vi "principal.vi"() -> ()   [LabVIEW 2010]
uses:
  <vilib>/addons/internet/NI_InternetTK_Common_VIs.lvlib
panel:
  out "status":bool
  out "Localizar Instrumento":u8(slide) scale=0.0..200.0
  out "Execução do ensaio":u8(slide) scale=0.0..100.0
  in  "inicio_time":string
  out "Contador_sim":bool
  out "Siave_sim":bool
  out "Excel._Workbook":refnum<k7>
  out "error out":errorcluster
  out "Excel._Worksheet":refnum<k7>
  in  "Tab k":T1(tab) caption="Tab Control 2"
  in  "Table 12000":string[][](table)
  in  "Table 20000":string[][](table)
  in  "Table 32000":string[][](table)
  in  "Table 40000":string[][](table)
  in  "Table 50000":string[][](table)
  in  "Table 65000":string[][](table)
  in  "Iniciar 2":bool
  in  "Iniciar":bool
  out "Rh %":dbl format="%.2g"
  out "Temp. ºC":dbl format="%.2g"
  in  "Patrimônio":string
  in  "Técnico executor":string
  out "k_list":i32[](array[numeric])=[1000, 2000, 4000, 8000, 15000, 40000]
  out "Vel_list":dbl[](array[numeric])
  out "nk * nVel":i32
  out "Serial disponivel":refnum<visa-resource-name>
  out "Velocidade":dbl
  out "Iteração atual":dbl
  out "Iterações":dbl
  out "Vmax":dbl
  out "Vmin":dbl
  out "k":dbl
  out "Freq. Atual":dbl format="%#.10g"
  out "Freq. Teórica":dbl format="%#.9g"
  out "Contador":bool
  out "Motover":bool
  # "Calibração do Motover"
  # "Equipamento Conectado"
  # "Parâmetros"
  # "Leitura Atual"
  # "simulação?"
  # "Identificação"
  # "Ensaio iniciado em:"
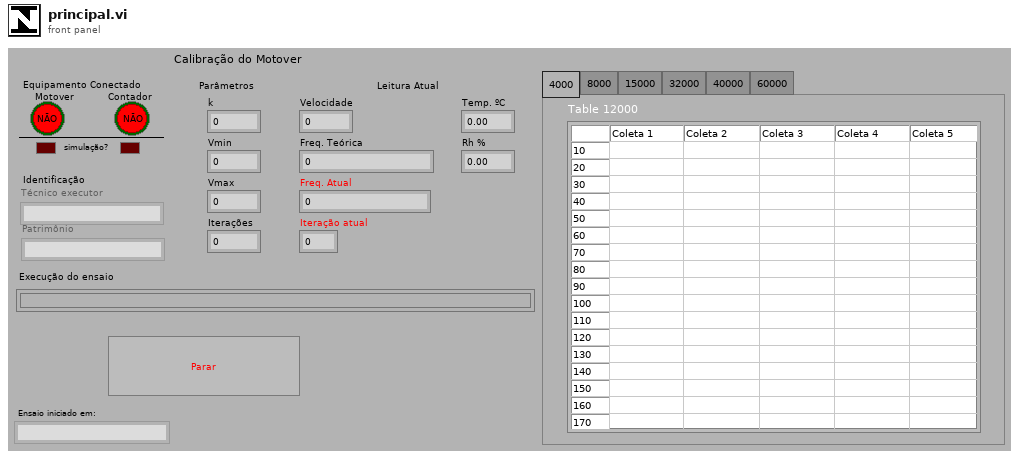
[diagram p1: front panel]
types:
  T1 = enum32{"4000", "8000", "15000", "32000", "40000", "60000"}
  T2 = enum8{"Enabled", "Disabled", "Disabled and Grayed Out"}
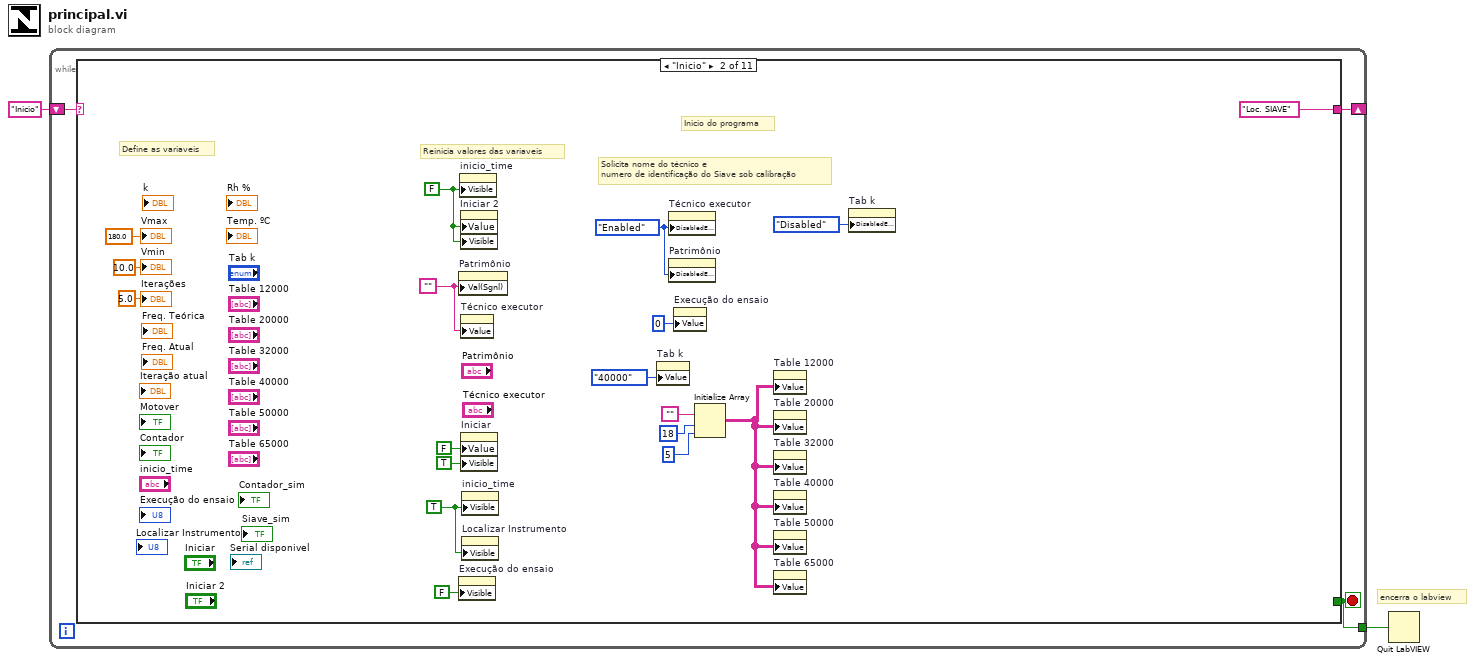
[diagram p0: block diagram]
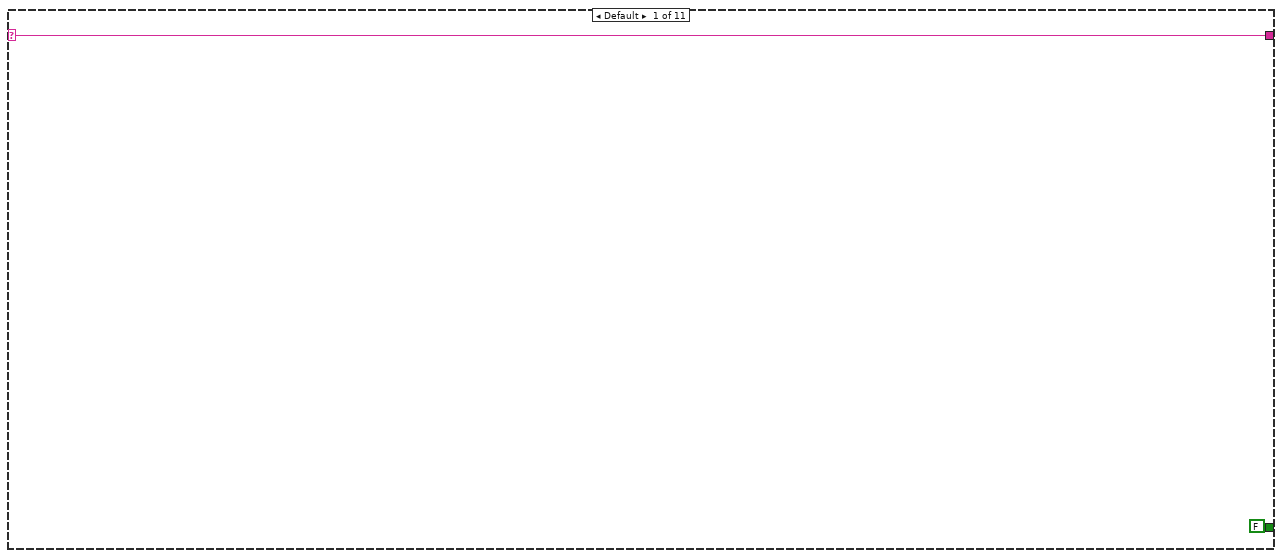
[diagram p2: hidden frame]
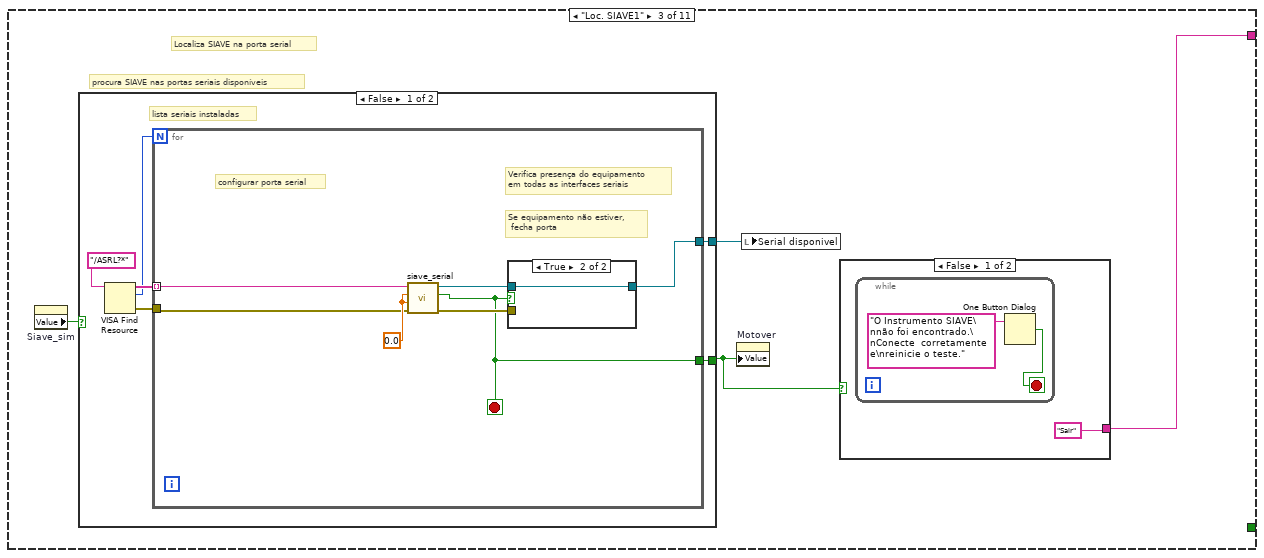
[diagram p3: hidden frame]
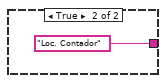
[diagram p4: hidden frame]
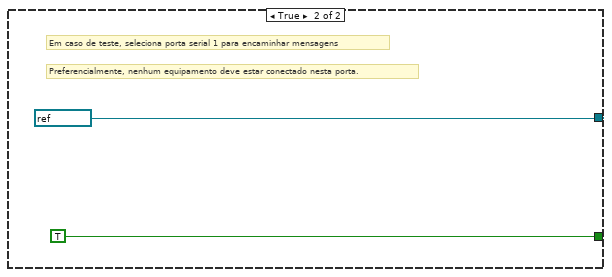
[diagram p6: hidden frame]
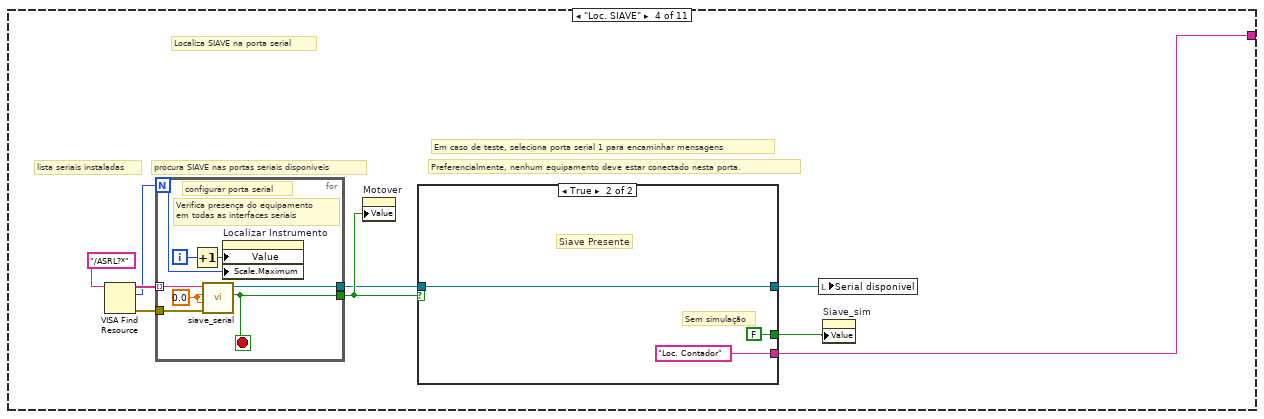
[diagram p7: hidden frame]
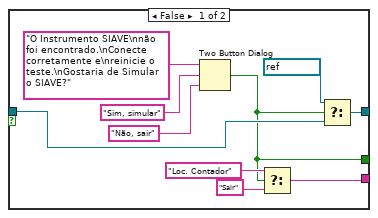
[diagram p8: hidden frame]
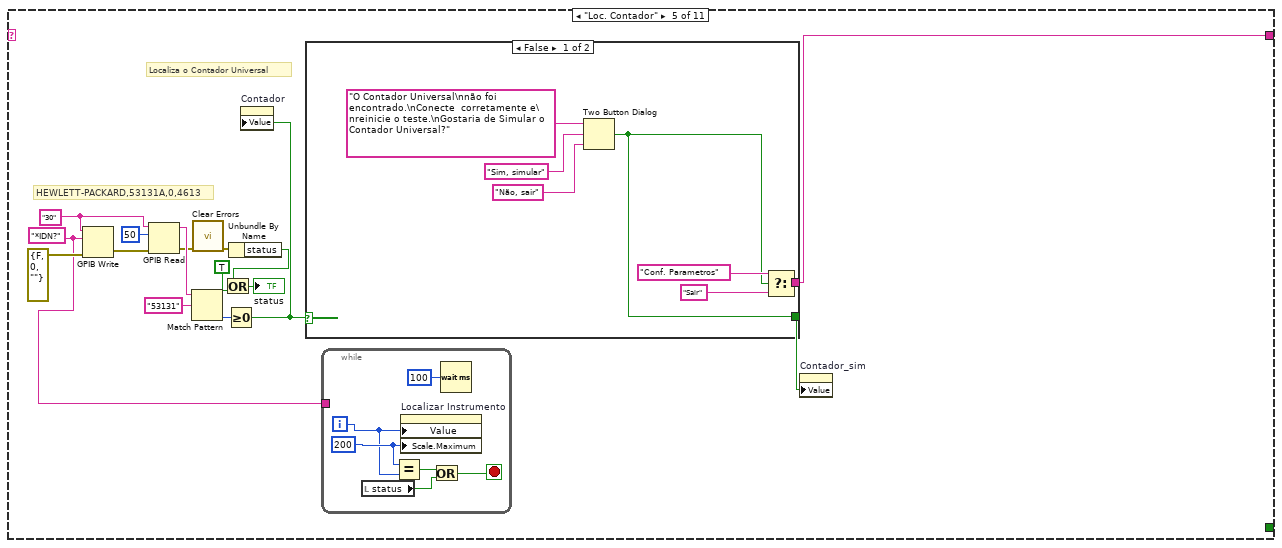
[diagram p9: hidden frame]
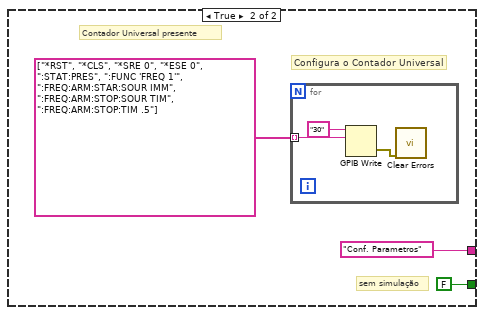
[diagram p10: hidden frame]
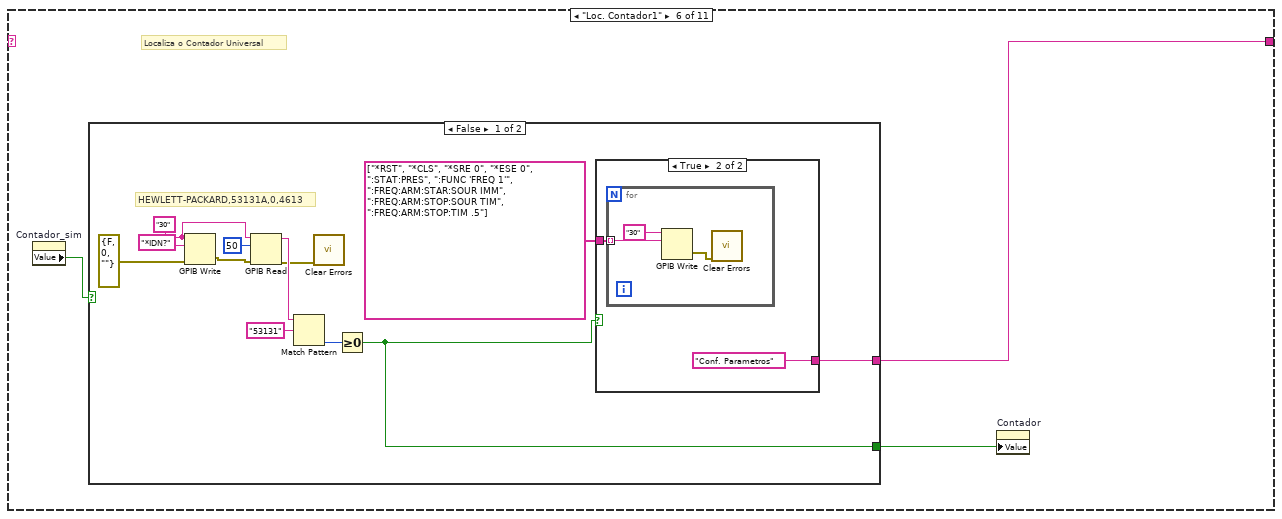
[diagram p11: hidden frame]
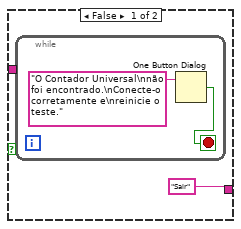
[diagram p12: hidden frame]
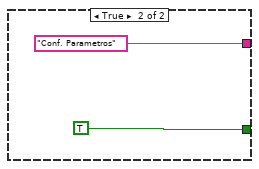
[diagram p13: hidden frame]
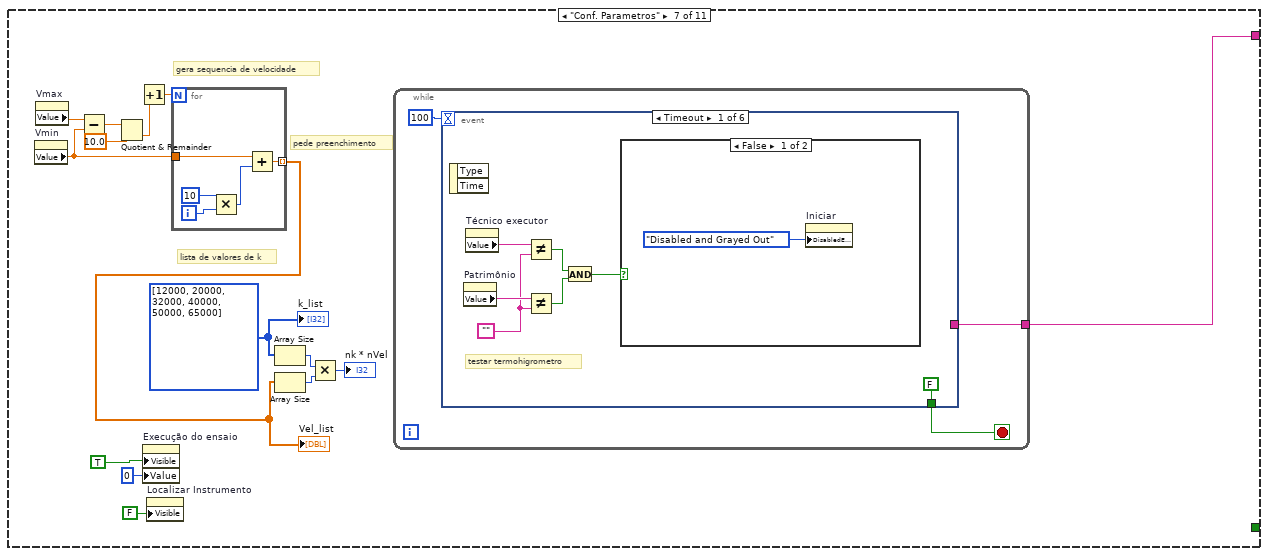
[diagram p14: hidden frame]
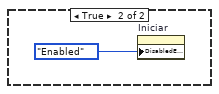
[diagram p15: hidden frame]
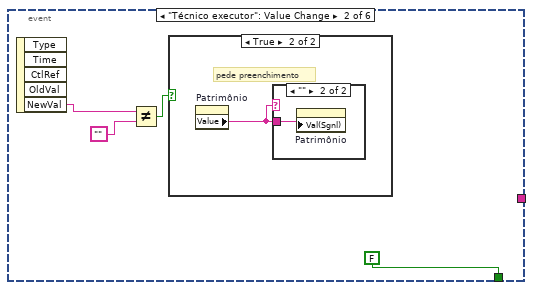
[diagram p16: hidden frame]
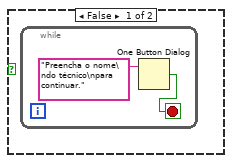
[diagram p17: hidden frame]
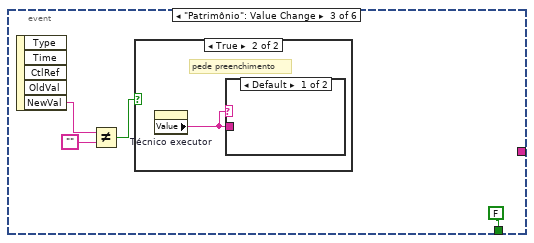
[diagram p19: hidden frame]
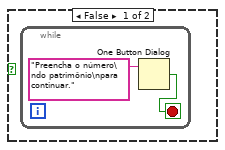
[diagram p20: hidden frame]
diagram:
  # "encerra o labview"
  n1 = while {
    shift-right: [w4] -> _
    shift-left: "Inicio" -> [w5]
    tunnel: [w3] -> w1
    stop <- w3 stop-if-true
    n2 = case shown="\"Inicio\"" w5 {
      selector: w5 -> [w6 _ _ _ _ _ _ _ _ _ _]
      tunnel: [FALSE _ _ _ _ _ _ _ _ _ TRUE] -> w3
      tunnel: [w6 "Loc. SIAVE" w27 w57 w85 w116 w143 "Coletar" w246 "Sair" "Sair"] -> w4
      frame Default {
      }
      frame "Inicio" {
        w9 = TRUE
        w20 = T2."Enabled" ("Disabled")
        w18 = FALSE ("Visible")
        w21 = ""
        # "Reinicia valores das variaveis"
        # "Solicita nome do técnico e\nnumero de identificação do Siave sob calibração"
        # "Define as variaveis"
        # "Inicio do programa"
        n3 = property on="Patrimônio" class="Str"("Val(Sgnl)"=w21) -> ()  [unwired: 2 in, 2 out]
        n4 = property on="Execução do ensaio" class="Slide (strict)"("Visible"=FALSE) -> ()  [unwired: 2 in, 2 out]
        n5 = property on="inicio_time" class="Str"("Visible"=w18) -> ()  [unwired: 2 in, 2 out]
        n6 = property on="Iniciar 2" class="Bool (strict)"("Value"=w18, "Visible"=w18) -> ()  [unwired: 2 in, 2 out]
        n7 = property on="Técnico executor" class="Str"("Value"=w21) -> ()  [unwired: 2 in, 2 out]
        n8 = property on="Iniciar" class="Bool (strict)"("Value"=FALSE ("Iniciar"), "Visible"=TRUE) -> ()  [unwired: 2 in, 2 out]
        n9 = property on="inicio_time" class="Str"("Visible"=w9) -> ()  [unwired: 2 in, 2 out]
        n10 = property on="Localizar Instrumento" class="Slide (strict)"("Visible"=w9) -> ()  [unwired: 2 in, 2 out]
        n11 = property on="Tab k" class="TabCtl (strict)"("Value"=T1."40000" ("Tab k")) -> ()  [unwired: 2 in, 2 out]
        n12 = property on="Técnico executor" class="Str"("DisabledEnum"=w20) -> ()  [unwired: 2 in, 2 out]
        n13 = property on="Patrimônio" class="Str"("DisabledEnum"=w20) -> ()  [unwired: 2 in, 2 out]
        n14 = property on="Execução do ensaio" class="Slide (strict)"("Value"=u8 0 ("Execução do ensaio")) -> ()  [unwired: 2 in, 2 out]
        n15 = Initialize Array("", 18, 5 ("dimension size")) -> (w12:string[][])
        n16 = property on="Table 12000" class="Tbl (strict)"("Value"=w12) -> ()  [unwired: 2 in, 2 out]
        n17 = property on="Table 20000" class="Tbl (strict)"("Value"=w12) -> ()  [unwired: 2 in, 2 out]
        n18 = property on="Table 32000" class="Tbl (strict)"("Value"=w12) -> ()  [unwired: 2 in, 2 out]
        n19 = property on="Table 40000" class="Tbl (strict)"("Value"=w12) -> ()  [unwired: 2 in, 2 out]
        n20 = property on="Table 50000" class="Tbl (strict)"("Value"=w12) -> ()  [unwired: 2 in, 2 out]
        n21 = property on="Table 65000" class="Tbl (strict)"("Value"=w12) -> ()  [unwired: 2 in, 2 out]
        n22 = property on="Tab k" class="TabCtl (strict)"("DisabledEnum"=T2."Disabled" ("Disabled")) -> ()  [unwired: 2 in, 2 out]
        "Vmin" <- 10.0 ("Vmin")
        "Vmax" <- 180.0 ("Vmax")
        "Iterações" <- 5.0 ("Iterações")
      }
      frame "Loc. SIAVE1" {
        # "procura SIAVE nas portas seriais disponíveis"
        # "Localiza SIAVE na porta serial"
        n23 = property on="Siave_sim" class="Bool (strict)"() -> ("Value"=w29:bool)  [unwired: 2 in, 2 out]
        n24 = case shown="False" w29 {
          tunnel: [w38 refnum<visa-resource-name> "COM1" ("VISA resource name out")] -> w26
          tunnel: [w37 TRUE] -> w28
          frame False {
            # "lista seriais instaladas"
            n25 = VISA Find Resource(11:"/ASRL?*" ("expression (\"?*\")")) -> (0:w35:errorcluster, 2:w34:u32, 3:w36:string[])  [unwired: 2 in]
            n26 = for {
              N: w34 -> [_]
              tunnel: w36 -> [w41] mode=indexing
              tunnel: [w45] -> w37
              tunnel: [w44] -> w38
              tunnel: w35 -> [w40]
              stop <- w45 stop-if-true
              w42 = 0.0 ("velocidade")
              # "Se equipamento não estiver,\n fecha porta"
              # "configurar porta serial"
              # "Verifica presença do equipamento\nem todas as interfaces seriais"
              n27 = call "siave_serial.vi"("error in (no error)"=w40, "velocidade"=w42, "k"=w42, "VISA resource name"=w41) -> ("error out"=w46:errorcluster, "ok"=w45:bool, "VISA resource name out"=w43:refnum<visa-resource-name>)  [unwired: 3 in, 2 out]
              n28 = case shown="True" w45 {
                tunnel: w43 -> [_ w47]
                tunnel: w46 -> [_ _]
                tunnel: [_ w47] -> w44
                frame False {
                }
                frame True {
                }
              }
            }
          }
          frame True {
            # "Preferencialmente, nenhum equipamento deve estar conectado nesta porta."
            # "Em caso de teste, seleciona porta serial 1 para encaminhar mensagens"
          }
        }
        n29 = property on="Motover" class="Bool (strict)"("Value"=w28) -> ()  [unwired: 2 in, 2 out]
        n30 = local write "Serial disponivel"(w26) -> ()
        n31 = case shown="False" w28 {
          tunnel: ["Sair" "Loc. Contador"] -> w27
          frame False {
            n32 = while {
              stop <- w31 stop-if-true
              n33 = One Button Dialog(message="O Instrumento SIAVE\nnão foi encontrado.\nConecte  corretamente e\nreinicie o teste.") -> (true=w31:bool)  [unwired: 1 in]
            }
          }
          frame True {
          }
        }
      }
      frame "Loc. SIAVE" {
        # "lista seriais instaladas"
        # "Preferencialmente, nenhum equipamento deve estar conectado nesta porta."
        # "Em caso de teste, seleciona porta serial 1 para encaminhar mensagens"
        # "procura SIAVE nas portas seriais disponíveis"
        # "Localiza SIAVE na porta serial"
        n34 = VISA Find Resource(11:"/ASRL?*" ("expression (\"?*\")")) -> (0:w54:errorcluster, 2:w53:u32, 3:w55:string[])  [unwired: 2 in]
        n35 = for {
          N: w53 -> [w61]
          tunnel: w55 -> [w64] mode=indexing
          tunnel: [w66] -> w58
          tunnel: [w62] -> w52
          tunnel: w54 -> [w63]
          i -> [w60]
          stop <- w66 stop-if-true
          w65 = 0.0 ("velocidade")
          # "configurar porta serial"
          # "Verifica presença do equipamento\nem todas as interfaces seriais"
          n36 = Increment(x=w60) -> (x+1=w59:i32)
          n37 = call "siave_serial.vi"("error in (no error)"=w63, "velocidade"=w65, "k"=w65, "VISA resource name"=w64) -> ("ok"=w66:bool, "VISA resource name out"=w62:refnum<visa-resource-name>)  [unwired: 3 in, 3 out]
          n38 = property on="Localizar Instrumento" class="Slide (strict)"("Value"=w59, "Scale.Maximum"=w61) -> ()  [unwired: 2 in, 2 out]
        }
        n39 = property on="Motover" class="Bool (strict)"("Value"=w58) -> ()  [unwired: 2 in, 2 out]
        n40 = case shown="True" w58 {
          tunnel: [w72 "Loc. Contador"] -> w57
          tunnel: w52 -> [w69 w78]
          tunnel: [w68 w78] -> w51
          tunnel: [w67 FALSE ("T button?")] -> w50
          frame False {
            n41 = Two Button Dialog(message="O Instrumento SIAVE\nnão foi encontrado.\nConecte  corretamente e\nreinicie o teste.\nGostaria de Simular o SIAVE?", 1:"Não, sair" ("F button name (\"Cancel\")"), 2:"Sim, simular" ("T button name (\"OK\")")) -> (T button?=w67:bool)
            n42 = Select(t="Loc. Contador", s=w67, f="Sair") -> (s? t:f=w72:string)
            n43 = Select(t=refnum<visa-resource-name> "COM1" ("VISA resource name out"), s=w67, f=w69) -> (s? t:f=w68:refnum<visa-resource-name>)
          }
          frame True {
            # "Sem simulação"
            # "Siave Presente"
          }
        }
        n44 = local write "Serial disponivel"(w51) -> ()
        n45 = property on="Siave_sim" class="Bool (strict)"("Value"=w50) -> ()  [unwired: 2 in, 2 out]
      }
      frame "Loc. Contador" {
        w94 = "30" ("address string")
        w84 = "*IDN?" ("data")
        # "HEWLETT-PACKARD,53131A,0,4613"
        # "Localiza o Contador Universal"
        n46 = GPIB Write(0:w94, 1:w84, 3:errorcluster {"status"=FALSE, "code"=0, "source"=""} ("error in")) -> (6:w95:errorcluster)  [unwired: 2 in, 1 out]
        n47 = GPIB Read(0:w94, 1:50 ("byte count"), 3:w95) -> (5:w91:string, 7:w88:errorcluster)  [unwired: 2 in, 1 out]
        n48 = Match Pattern(string=w91, regular expression="53131") -> (offset past match=w90:i32)  [unwired: 1 in, 3 out]
        n49 = call <vilib>:"Clear Errors.vi"("error in (no error)"=w88) -> ("error out"=w83:errorcluster)  [unwired: 6 in]
        n50 = Greater Or Equal To 0?(x=w90) -> (x >= 0?=w87:bool)
        n51 = Unbundle By Name(w83) -> ("status"=w80:bool)
        n52 = Or(x=w80, y=TRUE) -> (x .or. y?=→"status":bool)
        n53 = property on="Contador" class="Bool (strict)"("Value"=w87) -> ()  [unwired: 2 in, 2 out]
        n54 = case shown="False" w87 {
          tunnel: [w103 FALSE ("Contador_sim")] -> w86
          tunnel: [w102 "Conf. Parametros"] -> w85
          frame False {
            n55 = Two Button Dialog(message="O Contador Universal\nnão foi encontrado.\nConecte  corretamente e\nreinicie o teste.\nGostaria de Simular o Contador Universal?", 1:"Não, sair" ("F button name (\"Cancel\")"), 2:"Sim, simular" ("T button name (\"OK\")")) -> (T button?=w103:bool)
            n56 = Select(t="Conf. Parametros", s=w103, f="Sair") -> (s? t:f=w102:string)
          }
          frame True {
            # "Configura o Contador Universal"
            # "Contador Universal presente"
            # "sem simulação"
            n57 = for {
              tunnel: string[] ["*RST", "*CLS", "*SRE 0", "*ESE 0", ":STAT:PRES", ":FUNC 'FREQ 1'", ":FREQ:ARM:STAR:SOUR IMM", ":FREQ:ARM:STOP:SOUR TIM", ":FREQ:ARM:STOP:TIM .5"] -> [w114] mode=indexing
              n58 = GPIB Write(0:"30" ("address string"), 1:w114) -> (6:w112:errorcluster)  [unwired: 3 in, 1 out]
              n59 = call <vilib>:"Clear Errors.vi"("error in (no error)"=w112) -> ()  [unwired: 6 in, 1 out]
            }
          }
        }
        n60 = while {
          tunnel: w84 -> [_]
          i -> [w100]
          stop <- w97 stop-if-true
          w101 = 200
          n61 = local read "status"() -> (w96:bool)
          n62 = Equal?(x=w101, y=w100) -> (x = y?=w98:bool)
          n63 = property on="Localizar Instrumento" class="Slide (strict)"("Value"=w100, "Scale.Maximum"=w101) -> ()  [unwired: 2 in, 2 out]
          n64 = Or(x=w98, y=w96) -> (x .or. y?=w97:bool)
          n65 = Wait (ms)(milliseconds to wait=u32 100) -> ()  [unwired: 1 out]
        }
        n66 = property on="Contador_sim" class="Bool (strict)"("Value"=w86) -> ()  [unwired: 2 in, 2 out]
      }
      frame "Loc. Contador1" {
        # "Localiza o Contador Universal"
        n67 = property on="Contador_sim" class="Bool (strict)"() -> ("Value"=w115:bool)  [unwired: 2 in, 2 out]
        n68 = case shown="False" w115 {
          tunnel: [w121 TRUE] -> w117
          tunnel: [w119 "Conf. Parametros"] -> w116
          frame False {
            w127 = "30" ("address string")
            # "HEWLETT-PACKARD,53131A,0,4613"
            n69 = GPIB Write(0:w127, 1:"*IDN?" ("data"), 3:errorcluster {"status"=FALSE, "code"=0, "source"=""} ("error in")) -> (6:w128:errorcluster)  [unwired: 2 in, 1 out]
            n70 = GPIB Read(0:w127, 1:50 ("byte count"), 3:w128) -> (5:w123:string, 7:w118:errorcluster)  [unwired: 2 in, 1 out]
            n71 = Match Pattern(string=w123, regular expression="53131") -> (offset past match=w122:i32)  [unwired: 1 in, 3 out]
            n72 = call <vilib>:"Clear Errors.vi"("error in (no error)"=w118) -> ()  [unwired: 6 in, 1 out]
            n73 = Greater Or Equal To 0?(x=w122) -> (x >= 0?=w121:bool)
            n74 = case shown="True" w121 {
              tunnel: string[] ["*RST", "*CLS", "*SRE 0", "*ESE 0", ":STAT:PRES", ":FUNC 'FREQ 1'", ":FREQ:ARM:STAR:SOUR IMM", ":FREQ:ARM:STOP:SOUR TIM", ":FREQ:ARM:STOP:TIM .5"] -> [_ w134]
              tunnel: ["Sair" "Conf. Parametros"] -> w119
              frame False {
                n75 = while {
                  stop <- w131 stop-if-true
                  n76 = One Button Dialog(message="O Contador Universal\nnão foi encontrado.\nConecte-o  corretamente e\nreinicie o teste.") -> (true=w131:bool)  [unwired: 1 in]
                }
              }
              frame True {
                n77 = for {
                  tunnel: w134 -> [w137] mode=indexing
                  n78 = GPIB Write(0:"30" ("address string"), 1:w137) -> (6:w135:errorcluster)  [unwired: 3 in, 1 out]
                  n79 = call <vilib>:"Clear Errors.vi"("error in (no error)"=w135) -> ()  [unwired: 6 in, 1 out]
                }
              }
            }
          }
          frame True {
          }
        }
        n80 = property on="Contador" class="Bool (strict)"("Value"=w117) -> ()  [unwired: 2 in, 2 out]
      }
      frame "Conf. Parametros" {
        w146 = i32[] [12000, 20000, 32000, 40000, 50000, 65000]
        # "pede preenchimento"
        # "lista de valores de k"
        # "gera sequencia de velocidade"
        n81 = property on="Vmin" class="DigNum (strict)"() -> ("Value"=w152:dbl)  [unwired: 2 in, 2 out]
        n82 = property on="Vmax" class="DigNum (strict)"() -> ("Value"=w149:dbl)  [unwired: 2 in, 2 out]
        n83 = Subtract(x=w149, y=w152) -> (x-y=w150:dbl)
        n84 = Quotient & Remainder(x=w150, y=10.0) -> (floor(x/y)=w154:dbl)  [unwired: 1 out]
        n85 = Increment(x=w154) -> (x+1=w153:dbl)
        n86 = property on="Execução do ensaio" class="Slide (strict)"("Visible"=TRUE, "Value"=u8 0 ("Execução do ensaio")) -> ()  [unwired: 2 in, 2 out]
        n87 = property on="Localizar Instrumento" class="Slide (strict)"("Visible"=FALSE) -> ()  [unwired: 2 in, 2 out]
        n88 = for {
          N: w153 -> [_]
          tunnel: w152 -> [w205]
          tunnel: [w201] -> w145 mode=indexing
          i -> [w204]
          n89 = Multiply(x=10, y=w204) -> (x*y=w202:i32)
          n90 = Add(x=w205, y=w202) -> (x+y=w201:dbl)
        }
        "Vel_list" <- w145
        n91 = Array Size(array=w146) -> (size(s)=w148:i32)
        n92 = Array Size(array=w145) -> (size(s)=w147:i32)
        n93 = Multiply(x=w148, y=w147) -> (x*y=→"nk * nVel":i32)
        n94 = while {
          tunnel: [w155] -> w143
          stop <- w156 stop-if-true
          n95 = event shown="[0] Timeout" {
            selector: _ -> [_ _ _ _ _ _]
            dyn-events: _ -> [_ _ _ _ _ _]
            timeout: 100 -> [_ _ _ _ _ _]
            tunnel: [FALSE FALSE FALSE TRUE w195 _] -> w156
            tunnel: [_ _ _ "Excel" w194 "Loc. SIAVE"] -> w155
            event Timeout {
              w162 = ""
              # "testar termohigrometro"
              n96 = event-data() -> ()  [unwired: 1 in, 2 out]
              n97 = property on="Patrimônio" class="Str"() -> ("Value"=w163:string)  [unwired: 2 in, 2 out]
              n98 = property on="Técnico executor" class="Str"() -> ("Value"=w164:string)  [unwired: 2 in, 2 out]
              n99 = Not Equal?(x=w164, y=w162) -> (x != y?=w161:bool)
              n100 = Not Equal?(x=w163, y=w162) -> (x != y?=w160:bool)
              n101 = And(x=w161, y=w160) -> (x .and. y?=w159:bool)
              n102 = case shown="False" w159 {
                frame False {
                  n103 = property on="Iniciar" class="Bool (strict)"("DisabledEnum"=T2."Disabled and Grayed Out" ("Disabled")) -> ()  [unwired: 2 in, 2 out]
                }
                frame True {
                  n104 = property on="Iniciar" class="Bool (strict)"("DisabledEnum"=T2."Enabled" ("Disabled")) -> ()  [unwired: 2 in, 2 out]
                }
              }
            }
            event "Técnico executor": Value Change {
              n105 = event-data() -> ("NewVal"=w169:string)  [unwired: 1 in, 4 out]
              n106 = Not Equal?(x=w169, y="") -> (x != y?=w168:bool)
              n107 = case shown="True" w168 {
                frame False {
                  n108 = while {
                    stop <- w171 stop-if-true
                    n109 = One Button Dialog(message="Preencha o nome\ndo técnico\npara continuar.") -> (true=w171:bool)  [unwired: 1 in]
                  }
                }
                frame True {
                  # "pede preenchimento"
                  n110 = property on="Patrimônio" class="Str"() -> ("Value"=w173:string)  [unwired: 2 in, 2 out]
                  n111 = case shown="\"\"" w173 {
                    tunnel: w173 -> [_ w174]
                    frame Default {
                    }
                    frame "" {
                      n112 = property on="Patrimônio" class="Str"("Val(Sgnl)"=w174) -> ()  [unwired: 2 in, 2 out]
                    }
                  }
                }
              }
            }
            event "Patrimônio": Value Change {
              n113 = event-data() -> ("NewVal"=w178:string)  [unwired: 1 in, 4 out]
              n114 = Not Equal?(x=w178, y="") -> (x != y?=w176:bool)
              n115 = case shown="True" w176 {
                frame False {
                  n116 = while {
                    stop <- w179 stop-if-true
                    n117 = One Button Dialog(message="Preencha o número\ndo patrimônio\npara continuar.") -> (true=w179:bool)  [unwired: 1 in]
                  }
                }
                frame True {
                  # "pede preenchimento"
                  n118 = property on="Técnico executor" class="Str"() -> ("Value"=w181:string)  [unwired: 2 in, 2 out]
                  n119 = case shown="Default" w181 {
                    tunnel: w181 -> [_ w182]
                    frame Default {
                    }
                    frame "" {
                      n120 = property on="Técnico executor" class="Str"("Val(Sgnl)"=w182) -> ()  [unwired: 2 in, 2 out]
                    }
                  }
                }
              }
            }
            event "Iniciar": Mouse Up {
              w183 = TRUE ("Visible")
              w185 = T2."Disabled and Grayed Out" ("Disabled")
              # "muda botão: PARAR"
              # "quando pressionado, inicia coleta."
              n121 = event-data() -> ("CtlRef"=w191:refnum<vi>)  [unwired: 1 in, 6 out]
              n122 = property class="Bool (strict)"(reference=w191, "DisabledEnum"=T2."Enabled" ("Disabled"), "Visible"=FALSE) -> ()  [unwired: 1 in, 2 out]
              n123 = Get Date/Time In Seconds() -> (seconds since 1Jan1904=w188:timestamp)
              n124 = property on="inicio_time" class="Str"("Visible"=w183) -> ()  [unwired: 2 in, 2 out]
              n125 = property on="Iniciar 2" class="Bool (strict)"("Visible"=w183) -> ()  [unwired: 2 in, 2 out]
              n126 = To Double Precision Float(number=w188) -> (double precision float=w187:dbl)
              n127 = call <vilib>:"RFC-1123 Date.vi"("time (now)"=w187) -> ("GMT Date/Time"=w186:string)  [unwired: 1 in]
              n128 = property on="inicio_time" class="Str"("Value"=w186, "DisabledEnum"=w185) -> ()  [unwired: 2 in, 2 out]
              n129 = property on="Patrimônio" class="Str"("DisabledEnum"=w185) -> ()  [unwired: 2 in, 2 out]
              n130 = property on="Técnico executor" class="Str"("DisabledEnum"=w185) -> ()  [unwired: 2 in, 2 out]
            }
            event Panel Close? {
              w193 = "Sair"
              # "volta ao loop ao cancelar"
              # "incrementar saida com\nliberacao da porta serial\n\nao clicar no botão de encerrar"
              n131 = event-data() -> ()  [unwired: 1 in, 3 out]
              n132 = Two Button Dialog(message="Deseja encerrar o Ensaio?", 1:"Não" ("F button name (\"Cancel\")"), 2:"Sim" ("T button name (\"OK\")")) -> (T button?=w195:bool)
              n133 = Select(t=w193, s=w195, f=w193) -> (s? t:f=w194:string)
              n134 = event-data("Discard?"=TRUE) -> ()  [unwired: 1 in, 1 out]
            }
            event "Siave_sim", "Contador_sim": Value Change {
              n135 = event-data() -> ()  [unwired: 1 in, 5 out]
            }
          }
        }
        "k_list" <- w146
      }
      frame "Excel" {
        # "seleciona data (dd/mm/aaaa)"
        n136 = call "Open Excel and Make Visible.vi"("Visible Boolean"=TRUE) -> ("error out"=w218:errorcluster, "Excel._Application"=w214:refnum<k7>)  [unwired: 1 in]
        n137 = call <vilib>:"Application Directory.vi"() -> ("Application Directory"=w223:path)
        n138 = Build Path(base path=w223, name or relative path="data\\modelo_Calibração.xls") -> (appended path=w224:path)
        n139 = Path To String(path=w224) -> (string=w219:string)
        n140 = call "Open Specific WorkBook.vi"("error in (no error)"=w218, "Filename of Workbook"=w219, "Excel._Application"=w214) -> ("error out"=w220:errorcluster, "Excel._Workbook"=w212:refnum<k7>)
        "Excel._Workbook" <- w212
        n141 = call "Open Specific WorkSheet.vi"("error in (no error)"=w220, "Numeric"=1 ("planilha"), "Excel._Workbook"=w212) -> ("error out"=→"error out":errorcluster, "Excel._Worksheet"=→"Excel._Worksheet":refnum<k7>)
        n142 = property on="inicio_time" class="Str"() -> ("Value"=w209:string)  [unwired: 2 in, 2 out]
        n143 = property on="Técnico executor" class="Str"() -> ("Value"=w211:string)  [unwired: 2 in, 2 out]
        n144 = property on="Patrimônio" class="Str"() -> ("Value"=w210:string)  [unwired: 2 in, 2 out]
        n145 = property on="k_list" class="Arr (strict)"() -> ("Value"=w213:i32[])  [unwired: 2 in, 2 out]
        n146 = String Subset(string=w209, offset (0)=5, length (rest)=11 ("length (rest)")) -> (substring=w208:string)
        n147 = for {
          tunnel: w213 -> [_] mode=indexing
          tunnel: w212 -> [w239]
          tunnel: w208 -> [w228]
          tunnel: w211 -> [w227]
          tunnel: w210 -> [w226]
          i -> [w244]
          # "salva:\n- data\n- tecnico executor\n- patrimonio"
          # "seleciona pasta\nequivalente ao\nk atual"
          n148 = Increment(x=w244) -> (x+1=w242:i32)
          n149 = local read "error out"() -> (w243:errorcluster)
          n150 = call "Open Specific WorkSheet.vi"("error in (no error)"=w243, "Numeric"=w242, "Excel._Workbook"=w239) -> ("error out"=w241:errorcluster, "Excel._Worksheet"=w240:refnum<k7>)
          n151 = call "Set Cell Value with Range.vi"("Excel._Worksheet"=w240, "error in (no error)"=w241, "Value"=w228, "Col"=3, "Row"=8) -> ("error out"=w235:errorcluster, "Excel._Worksheet"=w234:refnum<k7>)  [unwired: 2 out]
          n152 = call "Set Cell Value with Range.vi"("Excel._Worksheet"=w234, "error in (no error)"=w235, "Value"=w227, "Col"=3, "Row"=9) -> ("error out"=w236:errorcluster, "Excel._Worksheet"=w233:refnum<k7>)  [unwired: 2 out]
          n153 = call "Set Cell Value with Range.vi"("Excel._Worksheet"=w233, "error in (no error)"=w236, "Value"=w226, "Col"=3, "Row"=10) -> ()  [unwired: 4 out]
        }
      }
      frame "Coletar" {
        # "freq=pulso/s = k(pulso/km)*vel(km/h)*1h/3600s"
        n154 = property on="k_list" class="Arr (strict)"() -> ("Value"=w248:i32[])  [unwired: 2 in, 2 out]
        n155 = property on="Vel_list" class="Arr (strict)"() -> ("Value"=w245:dbl[])  [unwired: 2 in, 2 out]
        n156 = for {
          tunnel: w248 -> [w255] mode=indexing
          shift-right: [w259] -> _
          shift-left: 0 -> [w260]
          tunnel: [w258] -> w246
          tunnel: w245 -> [w257]
          i -> [w252]
          stop <- w256 stop-if-true
          # "seleciona pasta\nequivalente ao\nk atual"
          n157 = local read "Excel._Workbook"() -> (w254:refnum<k7>)
          n158 = Increment(x=w252) -> (x+1=w253:i32)
          n159 = local read "error out"() -> (w249:errorcluster)
          n160 = call "Open Specific WorkSheet.vi"("error in (no error)"=w249, "Numeric"=w253, "Excel._Workbook"=w254) -> ("error out"=w250:errorcluster, "Excel._Worksheet"=w251:refnum<k7>)
          n161 = local write "Excel._Worksheet"(w251) -> ()
          n162 = for {
            N -> [w266]
            tunnel: w257 -> [w285] mode=indexing
            tunnel: w255 -> [w279]
            shift-right: [w286] -> w259
            shift-left: w260 -> [w270]
            tunnel: [w282] -> w258
            tunnel: [w280] -> w256
            tunnel: w251 -> [w263]
            tunnel: w250 -> [w262]
            i -> [w267]
            stop <- w280 stop-if-true
            n163 = Get Date/Time In Seconds() -> (seconds since 1Jan1904=w276:timestamp)
            n164 = Increment(x=w267) -> (x+1=w268:i32)
            n165 = property on="Siave_sim" class="Bool (strict)"() -> ("Value"=w281:bool)  [unwired: 2 in, 2 out]
            n166 = Equal To 0?(x=w267) -> (x = 0?=w265:bool)
            n167 = property on="k" class="DigNum (strict)"("Value"=w279) -> ()  [unwired: 2 in, 2 out]
            n168 = To Double Precision Float(number=w276) -> (double precision float=w275:dbl)
            n169 = Equal?(x=w266, y=w268) -> (x = y?=w264:bool)
            n170 = case shown="False" w281 {
              tunnel: w285 -> [w344 _]
              tunnel: w279 -> [w343 _]
              tunnel: [w342 TRUE ("ok")] -> w284
              tunnel: [w340 98.7 ("Umidade")] -> w277
              tunnel: [w339 120.3 ("Temp")] -> w278
              tunnel: [u32 500 ("milliseconds to wait") u32 0 ("milliseconds to wait")] -> w261
              frame False {
                n171 = property on="Serial disponivel" class="VISAName"() -> ("Value"=w341:refnum<visa-resource-name>)  [unwired: 2 in, 2 out]
                n172 = call "siave_serial.vi"("velocidade"=w344, "k"=w343, "VISA resource name"=w341) -> ("ok"=w342:bool, "Umidade"=w340:dbl, "Temp"=w339:dbl)  [unwired: 4 in, 2 out]
              }
              frame True {
              }
            }
            n173 = call <vilib>:"RFC-1123 Date.vi"("time (now)"=w275) -> ("GMT Date/Time"=w272:string)  [unwired: 1 in]
            n174 = String Subset(string=w272, offset (0)=17, length (rest)=8 ("length (rest)")) -> (substring=w271:string)
            n175 = Multiply(x=w279, y=w285) -> (x*y=w291:dbl)
            n176 = case shown="False" w265 {
              tunnel: w278 -> [w296 w337]
              tunnel: w277 -> [w297 w336]
              tunnel: w263 -> [w295 w335]
              tunnel: w262 -> [w294 w334]
              tunnel: w271 -> [w298 w333]
              tunnel: w270 -> [w293 w332]
              tunnel: [w293 w332] -> w269
              tunnel: w264 -> [w292 _]
              frame False {
                n177 = case shown="True" w292 {
                  tunnel: w298 -> [_ w317]
                  tunnel: w297 -> [_ w316]
                  tunnel: w296 -> [_ w315]
                  tunnel: w295 -> [_ w314]
                  tunnel: w294 -> [_ w313]
                  frame False {
                  }
                  frame True {
                    w300 = i16 2 ("precision (6)")
                    w299 = i16 2 ("precision (6)")
                    w305 = 6 ("Row")
                    # "se i=n salva fim"
                    # "Final"
                    n178 = Number To Fractional String(use system decimal point (T)=FALSE, number=w315, width (-)=w300, precision (6)=w300) -> (F-format string=w303:string)
                    n179 = call "Set Cell Value with Range.vi"("Excel._Worksheet"=w314, "error in (no error)"=w313, "Value"=w303, "Col"=w305, "Row"=12) -> ("error out"=w309:errorcluster, "Excel._Worksheet"=w310:refnum<k7>)  [unwired: 2 out]
                    n180 = Number To Fractional String(use system decimal point (T)=FALSE, number=w316, width (-)=w299, precision (6)=w299) -> (F-format string=w301:string)
                    n181 = call "Set Cell Value with Range.vi"("Excel._Worksheet"=w310, "error in (no error)"=w309, "Value"=w301, "Col"=w305, "Row"=13) -> ("error out"=w311:errorcluster, "Excel._Worksheet"=w312:refnum<k7>)  [unwired: 2 out]
                    n182 = call "Set Cell Value with Range.vi"("Excel._Worksheet"=w312, "error in (no error)"=w311, "Value"=w317, "Col"=w305, "Row"=14) -> ()  [unwired: 4 out]
                  }
                }
              }
              frame True {
                w319 = i16 2 ("precision (6)")
                w318 = i16 2 ("precision (6)")
                w324 = 5 ("Row")
                # "se i=0 salva ini"
                # "Inicio"
                n183 = Number To Fractional String(use system decimal point (T)=FALSE, number=w337, width (-)=w319, precision (6)=w319) -> (F-format string=w322:string)
                n184 = call "Set Cell Value with Range.vi"("Excel._Worksheet"=w335, "error in (no error)"=w334, "Value"=w322, "Col"=w324, "Row"=12) -> ("error out"=w328:errorcluster, "Excel._Worksheet"=w329:refnum<k7>)  [unwired: 2 out]
                n185 = Number To Fractional String(use system decimal point (T)=FALSE, number=w336, width (-)=w318, precision (6)=w318) -> (F-format string=w320:string)
                n186 = call "Set Cell Value with Range.vi"("Excel._Worksheet"=w329, "error in (no error)"=w328, "Value"=w320, "Col"=w324, "Row"=13) -> ("error out"=w330:errorcluster, "Excel._Worksheet"=w331:refnum<k7>)  [unwired: 2 out]
                n187 = call "Set Cell Value with Range.vi"("Excel._Worksheet"=w331, "error in (no error)"=w330, "Value"=w333, "Col"=w324, "Row"=14) -> ()  [unwired: 4 out]
              }
            }
            n188 = Divide(x=w291, y=3600.0) -> (x/y=w289:dbl)
            n189 = property on="Freq. Teórica" class="DigNum (strict)"("Value"=w289) -> ()  [unwired: 2 in, 2 out]
            n190 = Wait (ms)(milliseconds to wait=w261) -> ()  [unwired: 1 out]
            n191 = property on="Rh %" class="DigNum (strict)"("Value"=w277) -> ()  [unwired: 2 in, 2 out]
            n192 = property on="Temp. ºC" class="DigNum (strict)"("Value"=w278) -> ()  [unwired: 2 in, 2 out]
            n193 = property on="Motover" class="Bool (strict)"("Value"=w284) -> ()  [unwired: 2 in, 2 out]
            n194 = property on="nk * nVel" class="DigNum (strict)"() -> ("Value"=w283:i32)  [unwired: 2 in, 2 out]
            n195 = property on="Iterações" class="DigNum (strict)"() -> ("Value"=w288:dbl)  [unwired: 2 in, 2 out]
            n196 = Multiply(x=w288, y=w283) -> (x*y=w287:dbl)
            n197 = for {
              N: w288 -> [_]
              tunnel: w287 -> [w359]
              shift-right: [w356] -> w286
              shift-left: w269 -> [w358]
              tunnel: [w354] -> w282
              tunnel: [w353] -> w280
              tunnel: w267 -> [w351]
              i -> [w355]
              stop <- w353 stop-if-true
              n198 = Increment(x=w358) -> (x+1=w356:i32)
              n199 = event shown="[0] Timeout" {
                selector: _ -> [_ _ _]
                dyn-events: _ -> [_ _ _]
                timeout: 50 -> [_ _ _]
                tunnel: w355 -> [w372 _ _]
                tunnel: ["Salvar" w418 w426] -> w354
                tunnel: [FALSE ("T button?") w415 w423] -> w353
                tunnel: w351 -> [w368 _ _]
                event Timeout {
                  n200 = event-data() -> ()  [unwired: 1 in, 2 out]
                  n201 = property on="Contador_sim" class="Bool (strict)"() -> ("Value"=w367:bool)  [unwired: 2 in, 2 out]
                  n202 = Increment(x=w372) -> (x+1=w382:i32)
                  n203 = case shown="False" w367 {
                    tunnel: [w403 "2222.222225" ("data")] -> w360
                    tunnel: [w405 TRUE] -> w381
                    frame False {
                      w410 = "30" ("address string")
                      n204 = GPIB Write(0:w410, 1:"READ:FREQ?" ("data")) -> (6:w411:errorcluster)  [unwired: 3 in, 1 out]
                      n205 = GPIB Read(0:w410, 1:22 ("byte count"), 3:w411) -> (5:w403:string, 6:w408:bool[], 7:w404:errorcluster)  [unwired: 2 in]
                      n206 = Index Array(array=w408, index=15) -> (element=w406:bool)
                      n207 = Not(x=w406) -> (.not. x?=w405:bool)
                      n208 = call <vilib>:"Clear Errors.vi"("error in (no error)"=w404) -> ()  [unwired: 6 in, 1 out]
                    }
                    frame True {
                    }
                  }
                  n209 = property on="Iteração atual" class="DigNum (strict)"("Value"=w382) -> ()  [unwired: 2 in, 2 out]
                  n210 = Fract/Exp String To Number(use system decimal point (T)=FALSE, string=w360) -> (number=w365:dbl)  [unwired: 2 in, 1 out]
                  n211 = Number To Fractional String(use system decimal point (T)=FALSE, number=w365, precision (6)=i16 6) -> (F-format string=w361:string)  [unwired: 1 in]
                  n212 = property on="Contador" class="Bool (strict)"("Value"=w381) -> ()  [unwired: 2 in, 2 out]
                  n213 = Add(x=w372, y=3) -> (x+y=w371:i32)
                  n214 = property on="k" class="DigNum (strict)"() -> ("Value"=w376:dbl)  [unwired: 2 in, 2 out]
                  n215 = Fract/Exp String To Number(use system decimal point (T)=FALSE, string=w361) -> (number=w383:dbl)  [unwired: 2 in, 1 out]
                  n216 = local read "Excel._Worksheet"() -> (w374:refnum<k7>)
                  n217 = case shown="4000, Default" w376 {
                    tunnel: [w397 w398 w399 w400 w401 w402] -> w378
                    frame 4000, Default {
                      n218 = property on="Table 12000" class="Tbl (strict)"() -> ("Value"=w397:string[][])  [unwired: 2 in, 2 out]
                    }
                    frame 8000 {
                      n219 = property on="Table 20000" class="Tbl (strict)"() -> ("Value"=w398:string[][])  [unwired: 2 in, 2 out]
                    }
                    frame 15000 {
                      n220 = property on="Table 32000" class="Tbl (strict)"() -> ("Value"=w399:string[][])  [unwired: 2 in, 2 out]
                    }
                    frame 32000 {
                      n221 = property on="Table 40000" class="Tbl (strict)"() -> ("Value"=w400:string[][])  [unwired: 2 in, 2 out]
                    }
                    frame 40000 {
                      n222 = property on="Table 50000" class="Tbl (strict)"() -> ("Value"=w401:string[][])  [unwired: 2 in, 2 out]
                    }
                    frame 60000 {
                      n223 = property on="Table 65000" class="Tbl (strict)"() -> ("Value"=w402:string[][])  [unwired: 2 in, 2 out]
                    }
                  }
                  n224 = Add(x=w368, y=21) -> (x+y=w369:i32)
                  n225 = local read "error out"() -> (w375:errorcluster)
                  n226 = property on="Freq. Atual" class="DigNum (strict)"("Value"=w383) -> ()  [unwired: 2 in, 2 out]
                  n227 = Replace Array Subset(array=w378, new element=w361, index (row)=w368, index (col)=w372) -> (w377:string[][])
                  n228 = case shown="4000, Default" w376 {
                    tunnel: w377 -> [w386 w388 w390 w392 w394 w396]
                    tunnel: [T1."4000" ("Tab k") T1."8000" ("Tab k") T1."15000" ("Tab k") T1."32000" ("Tab k") T1."40000" ("Tab k") T1."60000" ("Tab k")] -> w366
                    frame 4000, Default {
                      n229 = property on="Table 12000" class="Tbl (strict)"("Value"=w386) -> ()  [unwired: 2 in, 2 out]
                    }
                    frame 8000 {
                      n230 = property on="Table 20000" class="Tbl (strict)"("Value"=w388) -> ()  [unwired: 2 in, 2 out]
                    }
                    frame 15000 {
                      n231 = property on="Table 32000" class="Tbl (strict)"("Value"=w390) -> ()  [unwired: 2 in, 2 out]
                    }
                    frame 32000 {
                      n232 = property on="Table 40000" class="Tbl (strict)"("Value"=w392) -> ()  [unwired: 2 in, 2 out]
                    }
                    frame 40000 {
                      n233 = property on="Table 50000" class="Tbl (strict)"("Value"=w394) -> ()  [unwired: 2 in, 2 out]
                    }
                    frame 60000 {
                      n234 = property on="Table 65000" class="Tbl (strict)"("Value"=w396) -> ()  [unwired: 2 in, 2 out]
                    }
                  }
                  n235 = call "Set Cell Value with Range.vi"("Excel._Worksheet"=w374, "error in (no error)"=w375, "Value"=w361, "Col"=w371, "Row"=w369) -> ()  [unwired: 4 out]
                  n236 = property on="Tab k" class="TabCtl (strict)"("Value"=w366) -> ()  [unwired: 2 in, 2 out]
                }
                event "Iniciar 2": Mouse Up {
                  n237 = event-data() -> ()  [unwired: 1 in, 7 out]
                  n238 = Two Button Dialog(message="Deseja encerrar o Ensaio?", 1:"Não" ("F button name (\"Cancel\")"), 2:"Sim" ("T button name (\"OK\")")) -> (T button?=w415:bool)
                  n239 = property on="Iniciar 2" class="Bool (strict)"("Value"=w415) -> ()  [unwired: 2 in, 2 out]
                  n240 = Select(t="Sair", s=w415, f="Salvar") -> (s? t:f=w418:string)
                }
                event Panel Close? {
                  # "isso não funcionou\n\no programa deixa de responder aos botoes,\nmas continua em execuçao"
                  n241 = event-data() -> ()  [unwired: 1 in, 3 out]
                  n242 = Two Button Dialog(message="Deseja encerrar o Ensaio?", 1:"Não" ("F button name (\"Cancel\")"), 2:"Sim" ("T button name (\"OK\")")) -> (T button?=w423:bool)
                  n243 = Select(t="Sair", s=w423, f="Salvar") -> (s? t:f=w426:string)
                  n244 = event-data("Discard?"=TRUE) -> ()  [unwired: 1 in, 1 out]
                }
              }
              n245 = Divide(x=w356, y=w359) -> (x/y=w349:dbl)
              n246 = Multiply(x=w349, y=100.0 ("x")) -> (x*y=w357:dbl)
              n247 = property on="Execução do ensaio" class="Slide (strict)"("Value"=w357) -> ()  [unwired: 2 in, 2 out]
            }
            "Velocidade" <- w285
          }
        }
      }
      frame "Salvar" {
        # "salva planilha com o nome definitivo"
        n248 = property on="Patrimônio" class="Str"() -> ("Value"=w438:string)  [unwired: 2 in, 2 out]
        n249 = call <vilib>:"Application Directory.vi"() -> ("Application Directory"=w440:path)
        n250 = Concatenate Strings("data\\Calibração_", w438, ".xls") -> (w436:string)
        n251 = Build Path(base path=w440, name or relative path=w436) -> (appended path=w435:path)
        n252 = local read "error out"() -> (w433:errorcluster)
        n253 = local read "Excel._Workbook"() -> (w434:refnum<k7>)
        n254 = Path To String(path=w435) -> (string=w432:string)
        n255 = invoke class="_Workbook" method="SaveAs"(reference=w434, error in=w433, "Filename"=w432, "Password"="siave") -> (reference out=w430:refnum<k7>)  [unwired: 11 in, 14 out]
        n256 = local write "Excel._Workbook"(w430) -> ()
      }
      frame "Sair" {
        n257 = property on="Serial disponivel" class="VISAName"() -> ("Value"=w448:refnum<visa-resource-name>)  [unwired: 2 in, 2 out]
        n258 = property on="Siave_sim" class="Bool (strict)"() -> ("Value"=w447:bool)  [unwired: 2 in, 2 out]
        n259 = local read "Excel._Workbook"() -> (w446:refnum<k7>)
        n260 = local read "error out"() -> (w445:errorcluster)
        n261 = case shown="True" w447 {
          tunnel: w448 -> [w458 _]
          frame False {
            w457 = 0.0 ("k")
            # "desliga gerador"
            n262 = call "siave_serial.vi"("velocidade"=w457, "k"=w457, "VISA resource name"=w458) -> ()  [unwired: 4 in, 5 out]
          }
          frame True {
          }
        }
        n263 = property class="_Workbook"(reference=w446, error in=w445) -> (reference out=w444:refnum<k7>, error out=w442:errorcluster, "HasPassword"=w443:bool)
        n264 = case shown="No Error" w442 {
          tunnel: w444 -> [w453 _]
          tunnel: w442 -> [w452 _]
          tunnel: w443 -> [w451 _]
          frame No Error {
            n265 = case shown="False" w451 {
              tunnel: w452 -> [w455 _]
              tunnel: w453 -> [w454 _]
              frame False {
                # "fecha arquivo de template"
                n266 = invoke class="_Workbook" method="Close"(reference=w454, error in=w455, "SaveChanges"=FALSE) -> ()  [unwired: 3 in, 6 out]
              }
              frame True {
                # "mantem aberta a planilha\npara inspecao do \noperador"
              }
            }
          }
          frame Error {
          }
        }
      }
    }
  }
  n267 = Quit LabVIEW(quit? (T)=w1) -> ()
